vi "Item_OnPopupMenu.vi"(11 "Object":T1) -> ()   [LabVIEW 2020, in "Project Provider.lvlib"]
uses:
  Project Provider.lvlib
  <resource>/Framework/Providers/API/mxLvMenuItem.ctl
  <resource>/Framework/Providers/API/ItemRef.ctl
panel:
  out "error out":errorcluster
  in  "error in":errorcluster
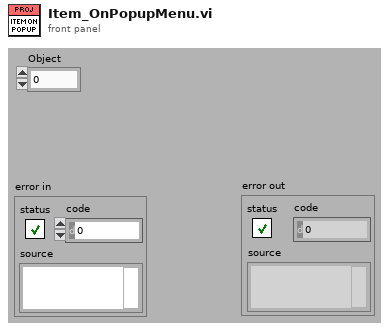
[diagram p1: front panel]
types:
  T1 = typedef "ItemRef.ctl" = u64
  T2 = typedef "mxLvMenuItem.ctl" = cluster{"Menu Name":string, "Description":string, "Icon File Name":path, "Menu Tag":string, "Enabled":bool, "Checked":bool, "Separator":bool, "Batchable":bool, "Weight":i32, "Batch Mode (Ignored if Not Batchable)":enum32{"Show If All Items Support Command", "Show If Any Items Support Command"}, "Menu Location":enum32{"<None>", "Project", "Project / Build Specifications", "Tools", "Tools / Source Control", "Tools / Real-Time Module", "Help"}, "Exclude From Getting Started Window Menu":bool}
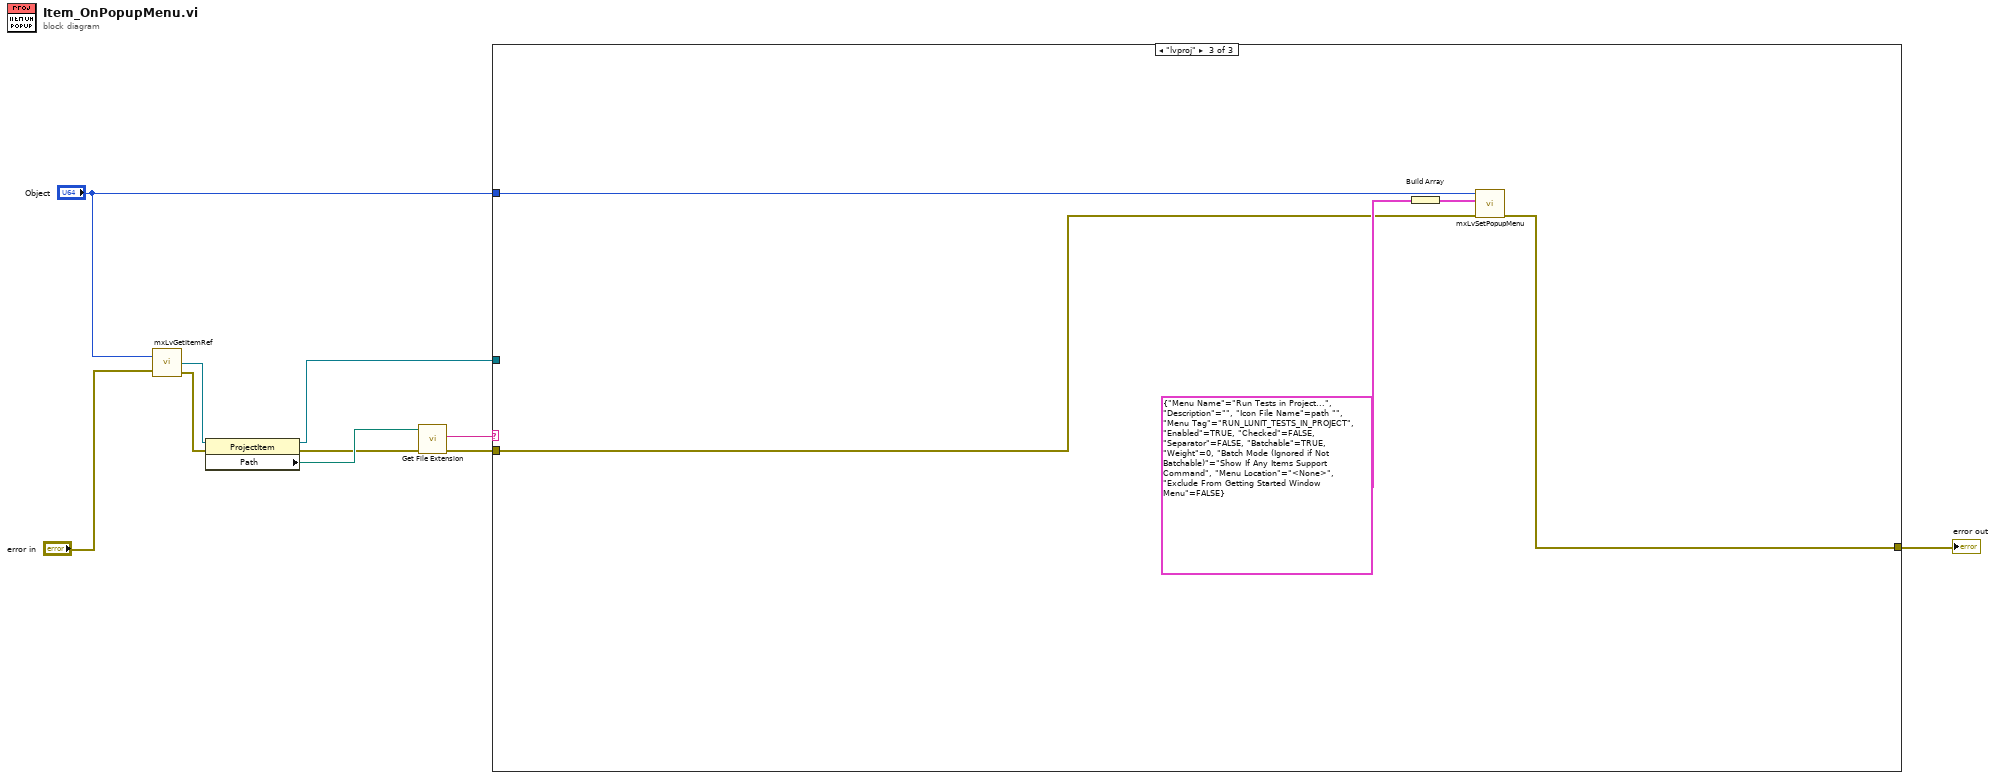
[diagram p0: block diagram]
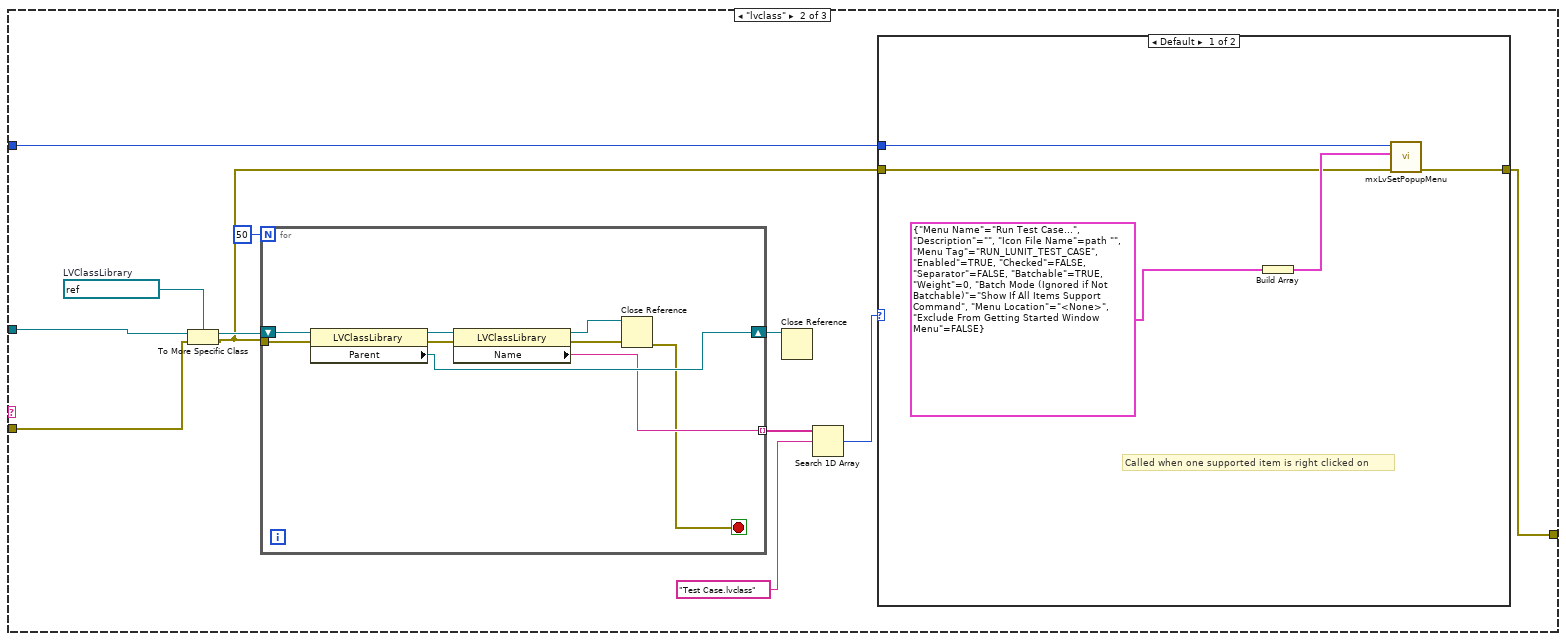
[diagram p3: hidden frame]
diagram:
  n1 = call <resource>:"mxLvGetItemRef.vi"("Item"="Object", "error in"="error in") -> ("Item Refnum"=w4:refnum<vi>, "error out"=w5:errorcluster)  [unwired: 1 out]
  n2 = property class="ProjectItem"(reference=w4, error in=w5) -> (reference out=w3:refnum<vi>, error out=w6:errorcluster, "Path"=w7:path)
  n3 = call <vilib>:"Get File Extension.vi"("error in (no error)"=w6, "file"=w7) -> ("error out"=w2:errorcluster, "lowercase file extension"=w1:string)  [unwired: 5 in, 3 out]
  n4 = case shown="\"lvproj\"" w1 {
    tunnel: [w11 w23 w42] -> w10
    tunnel: "Object" -> [_ w22 w43]
    tunnel: w2 -> [w11 w13 w39]
    tunnel: w3 -> [_ w14 _]
    frame Default {
    }
    frame "lvclass" {
      w16 = refnum<vi> refnum  # LVClassLibrary
      n5 = To More Specific Class(target class=w16, reference=w14, error in=w13) -> (specific class reference=w15:refnum<vi>, error out=w12:errorcluster)
      n6 = for {
        N: 50 -> [_]
        tunnel: w12 -> [w31]
        shift-right: [w30] -> w21
        shift-left: w15 -> [w32]
        tunnel: [w29] -> w18 mode=indexing
        stop <- w28 stop-if-true
        n7 = property class="LVClassLibrary"(reference=w32, error in=w31) -> (reference out=w27:refnum<vi>, error out=w25:errorcluster, "Parent"=w30:refnum<vi>)
        n8 = property class="LVClassLibrary"(reference=w27, error in=w25) -> (reference out=w26:refnum<vi>, error out=w24:errorcluster, "Name"=w29:string)
        n9 = Close Reference(reference=w26, error in (no error)=w24) -> (error out=w28:errorcluster)
      }
      n10 = Close Reference(reference=w21) -> ()  [unwired: 1 in, 1 out]
      n11 = Search 1D Array(1D array=w18, element="Test Case.lvclass") -> (index of element=w19:i32)  [unwired: 1 in]
      n12 = case shown="Default" w19 {
        tunnel: [w37 w38] -> w23
        tunnel: w22 -> [w36 _]
        tunnel: w12 -> [w33 w38]
        frame Default {
          # "Called when one supported item is right clicked on"
          n13 = Build Array(T2 {"Menu Name"="Run Test Case...", "Description"="", "Icon File Name"=path "", "Menu Tag"="RUN_LUNIT_TEST_CASE", "Enabled"=TRUE, "Checked"=FALSE, "Separator"=FALSE, "Batchable"=TRUE, "Weight"=0, "Batch Mode (Ignored if Not Batchable)"=enum."Show If All Items Support Command", "Menu Location"=enum."<None>", "Exclude From Getting Started Window Menu"=FALSE} ("Menu Item")) -> (w35:T2[])
          n14 = call <resource>:"mxLvSetPopupMenu.vi"("error in"=w33, "Popup Menu Items"=w35, "Item"=w36) -> ("error out"=w37:errorcluster)  [unwired: 7 in, 1 out]
        }
        frame -1 {
        }
      }
    }
    frame "lvproj" {
      n15 = Build Array(T2 {"Menu Name"="Run Tests in Project...", "Description"="", "Icon File Name"=path "", "Menu Tag"="RUN_LUNIT_TESTS_IN_PROJECT", "Enabled"=TRUE, "Checked"=FALSE, "Separator"=FALSE, "Batchable"=TRUE, "Weight"=0, "Batch Mode (Ignored if Not Batchable)"=enum."Show If Any Items Support Command", "Menu Location"=enum."<None>", "Exclude From Getting Started Window Menu"=FALSE} ("Menu Item")) -> (w41:T2[])
      n16 = call <resource>:"mxLvSetPopupMenu.vi"("error in"=w39, "Popup Menu Items"=w41, "Item"=w43) -> ("error out"=w42:errorcluster)  [unwired: 7 in, 1 out]
    }
  }
  "error out" <- w10
